vi "__uintComparisons.vi"(9 "Timeout (-1)":T1=-1, 10 "Uint2 in":u8[](array[numeric])=[0], 11 "Uint1 in":u8[](array[numeric])=[0]) -> (0 "Timing comparison":u32, 1 "Timeout":bool, 2 "Uint1 != Uint2":bool, 3 "Uint1 = Uint2":bool, 4 "Uint1 <= Uint2":bool, 5 "Uint1 > Uint2":bool, 6 "Uint1 >= Uint2":bool, 7 "Uint1 < Uint2":bool)   [LabVIEW 2011, in "UintClass.lvclass"]
uses:
  UintClass.lvclass
  timeout.ctl
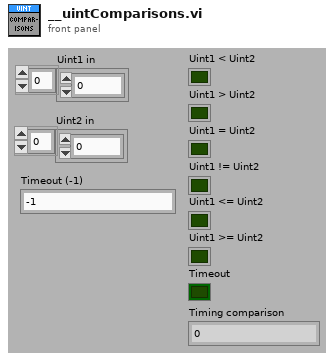
[diagram p1: front panel]
types:
  T1 = typedef "UintClass.lvclass/timeout.ctl" = i32
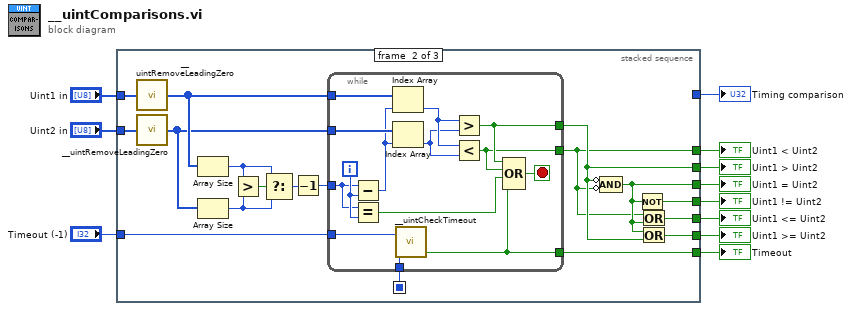
[diagram p0: block diagram]
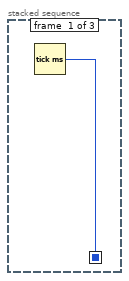
[diagram p2: hidden frame]
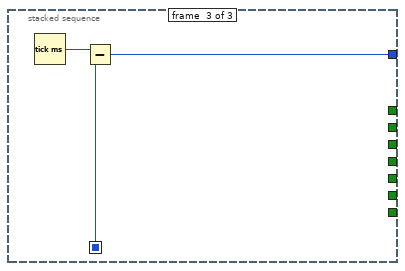
[diagram p3: hidden frame]
diagram:
  n1 = stacked-sequence {
    seq-local: [w12 _ _] -> [_ w15 w46]
    tunnel: "Uint2 in" -> [_ w30 _]
    tunnel: "Uint1 in" -> [_ w29 _]
    tunnel: [_ w28 _] -> w9
    tunnel: [_ w27 _] -> w8
    tunnel: [_ w26 _] -> w7
    tunnel: [_ w25 _] -> w6
    tunnel: [_ w24 _] -> w5
    tunnel: [_ w23 _] -> w4
    tunnel: "Timeout (-1)" -> [_ w14 _]
    tunnel: [_ _ w45] -> w2
    tunnel: [_ w13 _] -> w1
    frame #0 {
      n2 = Tick Count (ms)() -> (millisecond timer value=w12:u32)
    }
    frame #1 {
      n3 = call "__uintRemoveLeadingZero.vi"("Uint in"=w29) -> ("Uint out"=w17:u8[])
      n4 = call "__uintRemoveLeadingZero.vi"("Uint in"=w30) -> ("Uint out"=w16:u8[])
      n5 = Array Size(array=w17) -> (size(s)=w20:i32)
      n6 = Array Size(array=w16) -> (size(s)=w21:i32)
      n7 = Greater?(x=w20, y=w21) -> (0:w19:bool)
      n8 = Select(t=w20, s=w19, f=w21) -> (s? t:f=w22:i32)
      n9 = Decrement(x=w22) -> (x-1=w18:i32)
      n10 = while {
        tunnel: w17 -> [w44]
        tunnel: w16 -> [w43]
        tunnel: [w38] -> w28
        tunnel: w18 -> [w41]
        tunnel: [w37] -> w25
        tunnel: w15 -> [w33]
        tunnel: w14 -> [w32]
        tunnel: [w31] -> w13
        i -> [w42]
        stop <- w34 stop-if-true
        n11 = Subtract(x=w41, y=w42) -> (x-y=w35:i32)
        n12 = Equal?(x=w41, y=w42) -> (x = y?=w36:bool)
        n13 = Index Array(array=w44, index=w35) -> (element=w40:u8)
        n14 = Index Array(array=w43, index=w35) -> (element=w39:u8)
        n15 = call "__uintCheckTimeout.vi"("Millisecond timer value"=w33, "Timeout (-1)"=w32) -> ("Timeout?"=w31:bool)
        n16 = Greater?(x=w40, y=w39) -> (0:w38:bool)
        n17 = Less?(x=w40, y=w39) -> (x < y?=w37:bool)
        n18 = Compound Arithmetic op=OR(w38, w37, w36, w31) -> (w34:bool)
      }
      n19 = Compound Arithmetic op=AND(invert w28, invert w25) -> (w27:bool)
      n20 = Not(x=w27) -> (.not. x?=w23:bool)
      n21 = Or(x=w25, y=w27) -> (x .or. y?=w24:bool)
      n22 = Or(x=w27, y=w28) -> (x .or. y?=w26:bool)
    }
    frame #2 {
      n23 = Tick Count (ms)() -> (millisecond timer value=w47:u32)
      n24 = Subtract(x=w47, y=w46) -> (x-y=w45:u32)
    }
  }
  "Uint1 > Uint2" <- w9
  "Uint1 = Uint2" <- w8
  "Uint1 >= Uint2" <- w7
  "Uint1 < Uint2" <- w6
  "Uint1 <= Uint2" <- w5
  "Uint1 != Uint2" <- w4
  "Timing comparison" <- w2
  "Timeout" <- w1
